vi "LS372_manual_heater_output.vi"(4 "Heater Resistance":dbl, 5 "Heater Power":dbl format="%#_5f", 6 "Manuel Heater":bool, 7 "VISA-Ressourcenname":refnum<visa-resource-name>) -> ()   [LabVIEW 2018]
uses:
  Equipment/Lake Shore 372/Lake Shore 372.lvlib
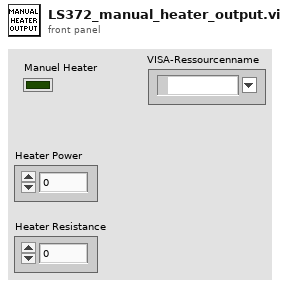
[diagram p1: front panel]
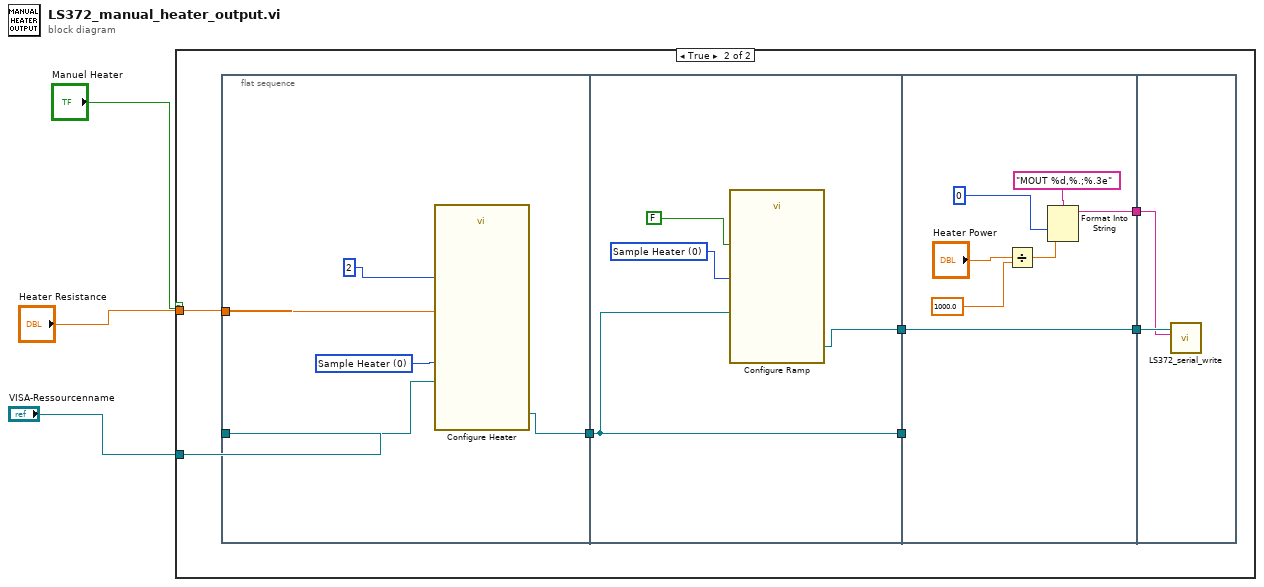
[diagram p0: block diagram]
diagram:
  n1 = case shown="True" "Manuel Heater" {
    tunnel: "VISA-Ressourcenname" -> [_ w5]
    tunnel: "Heater Resistance" -> [_ w4]
    frame False {
    }
    frame True {
      n2 = flat-sequence {
        tunnel: w5 -> [w15]
        tunnel: [w14] -> w10
        tunnel: w4 -> [w12]
        tunnel: [w19] -> w9
        tunnel: w10 -> [w19]
        tunnel: [w18] -> w8
        tunnel: w9 -> [_]
        tunnel: w8 -> [w21]
        tunnel: [w21] -> w7
        tunnel: [w20] -> w6
        tunnel: w7 -> [w28]
        tunnel: w6 -> [w27]
        frame #0 {
          w13 = u16 0 items=["Sample Heater ", "Warm-up Heater "] ("Output (0: Sample Heater)")
          n3 = call "Configure Heater.vi"("VISA resource name"=w15, "Current Power (1: Current)"=u16 2, "Output (0: Sample Heater)"=w13, "Heater Resistance Load (50 ohms)"=w12) -> ("VISA resource name out"=w14:refnum<visa-resource-name>)  [unwired: 10 in, 1 out]
        }
        frame #1 {
          w17 = u16 0 items=["Sample Heater ", "Warm-up Heater "] ("Output (0: Sample Heater)")
          n4 = call "Configure Ramp.vi"("Enable Ramping (F: Disable)"=FALSE, "Output (0: Sample Heater)"=w17, "VISA resource name"=w19) -> ("VISA resource name out"=w18:refnum<visa-resource-name>)  [unwired: 7 in, 1 out]
        }
        frame #2 {
          n5 = Divide(x="Heater Power", y=1000.0) -> (x/y=w25:dbl)
          n6 = Format Into String(format string="MOUT %d,%.;%.3e", u16 0, w25) -> (resulting string=w20:string)  [unwired: 2 in, 1 out]
        }
        frame #3 {
          n7 = call "LS372_serial_write.vi"("Write Buffer (\"\")"=w27, "VISA resource name"=w28) -> ()  [unwired: 7 in, 3 out]
        }
      }
    }
  }
